vi "Channel Page.vi"(8 "error in (no error)":errorcluster, 11 "Node Ptr":T1 format="%.0x") -> (0 "error out":errorcluster)   [LabVIEW 2009, in "NI-XNET Custom Device.lvlib"]
uses:
  NI-XNET Custom Device.lvlib
  <vilib>/NI VeriStand/Custom Device API/Custom Device Item Ref.ctl
  <vilib>/NI VeriStand/Custom Device API/Get Item Property (Variant).vi
  <vilib>/NI VeriStand/Custom Device API/Custom Device API.lvlib
  Program Files/National Instruments/LabVIEW 2009/resource/objmgr/xnet.rc
panel:
  out "Name":string
  out "Unit":string
  out "Start Bit":u32
  out "Scaling Offset":dbl
  out "Scaling Factor":dbl
  out "Number of Bits":u32
  out "Minimum Value":dbl
  out "Maximum Value":dbl
  out "Default Value":dbl
  out "Data Type":u32(ring) items=["Signed", "Unsigned", "IEEE Float"]
  out "Comment":string
  out "Byte Order":u32(ring) items=["Little Endian", "Big Endian"]
  in  "Header":cluster{"Section Name":string}={"Section Name"="Signal Properties"}
  in  "Delete":bool
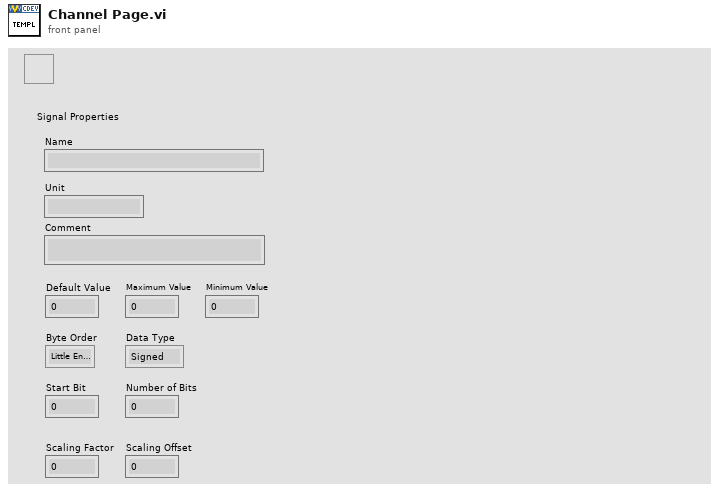
[diagram p1: front panel]
types:
  T1 = typedef "Custom Device API.lvlib/Custom Device Item Ref.ctl" = u64
  T2 = typedef "Custom Device API.lvlib/Custom Device Commands.ctl" = enum16{"Default", "Item renamed", "Shutdown"}
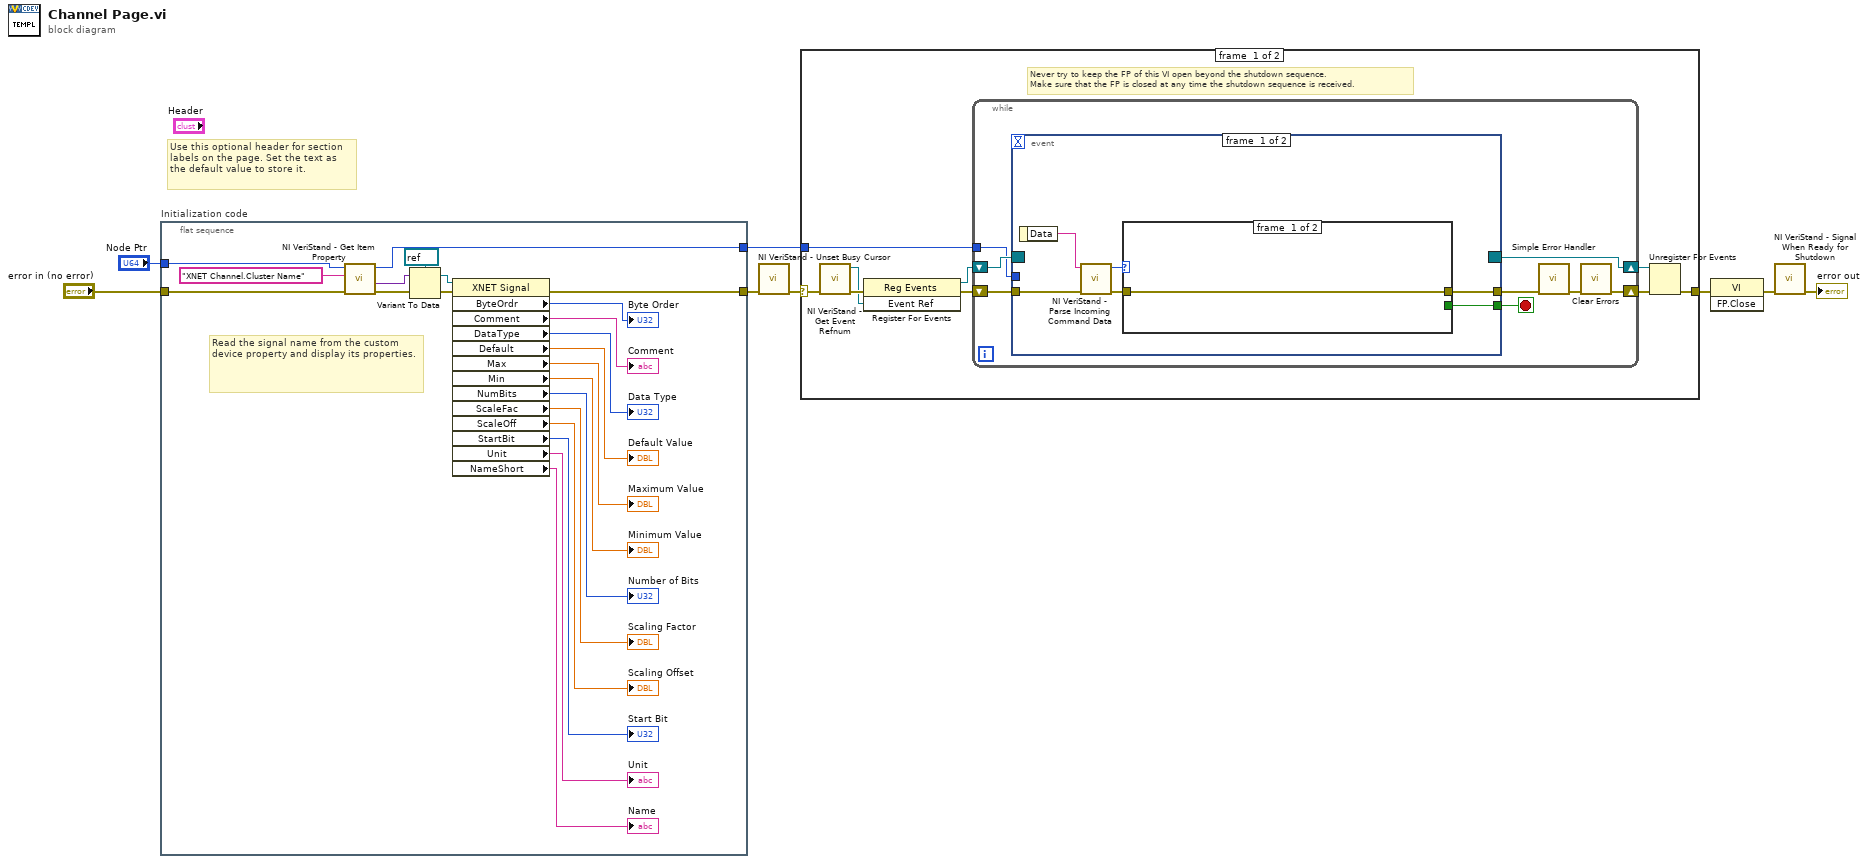
[diagram p0: block diagram]
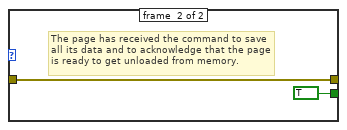
[diagram p2: hidden frame]
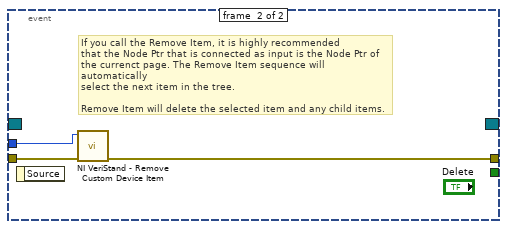
[diagram p3: hidden frame]
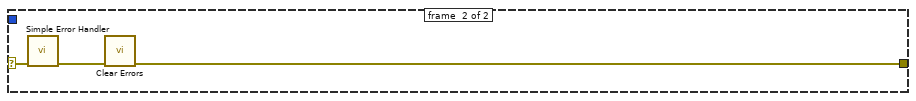
[diagram p4: hidden frame]
diagram:
  # "Use this optional header for section labels on the page. Set the text as the default value to store it."
  n1 = flat-sequence "Initialization code" {
    tunnel: "error in (no error)" -> [w12]
    tunnel: "Node Ptr" -> [w11]
    tunnel: [w24] -> w4
    tunnel: [w10] -> w1
    frame #0 {
      # "Read the signal name from the custom device property and display its properties."
      n2 = call-poly <vilib>:"NI VeriStand - Get Item Property.vi"("error in (no error)"=w12, "Property Name"="XNET Channel.Cluster Name", "Item Ref in"=w11) -> ("error out"=w25:errorcluster, "Value"=w28:variant, "Item Ref out"=w10:T1)  [unwired: 5 in, 1 out]
      n3 = Variant To Data(error in=w25, Variant=w28, type=refnum<k21> refnum ("XNET Signal Constant")) -> (error out=w26:errorcluster, data=w27:refnum<k21>)
      n4 = property class="XNET Signal"(reference=w27, error in=w26) -> (error out=w24:errorcluster, "ByteOrdr"=→"Byte Order":u32, "Comment"=→"Comment":string, "DataType"=→"Data Type":u32, "Default"=→"Default Value":dbl, "Max"=→"Maximum Value":dbl, "Min"=→"Minimum Value":dbl, "NumBits"=→"Number of Bits":u32, "ScaleFac"=→"Scaling Factor":dbl, "ScaleOff"=→"Scaling Offset":dbl, "StartBit"=→"Start Bit":u32, "Unit"=→"Unit":string, "NameShort"=→"Name":string)  [unwired: 1 out]
    }
  }
  n5 = call <vilib>:"NI VeriStand - Unset Busy Cursor.vi"("error in (no error)"=w4) -> ("error out"=w3:errorcluster)  [unwired: 10 out]
  n6 = case shown="No Error" w3 {
    selector: w3 -> [w32 w62]
    tunnel: [w36 w60] -> w8
    tunnel: w1 -> [w31 _]
    frame #0 {
      # "Never try to keep the FP of this VI open beyond the shutdown sequence.\nMake sure that the FP is closed at any time the shutdown sequence is received."
      n7 = call <vilib>:"NI VeriStand - Get Event Refnum.vi"("error in (no error)"=w32) -> ("error out"=w39:errorcluster, "Event Ref"=w35:refnum<user-event>)  [unwired: 9 out]
      n8 = register-events(error in=w39, w35) -> (reference out=w33:refnum<event-registration>, error out=w34:errorcluster)  [unwired: 1 in]
      n9 = while {
        shift-right: [w41] -> w37
        shift-left: w34 -> [w46]
        shift-right: [w47] -> w38
        shift-left: w33 -> [w45]
        tunnel: w31 -> [w40]
        stop <- w44 stop-if-true
        n10 = event shown="[1] \"Delete\": Value Change" {
          selector: w45 -> [_ _]
          dyn-events: [_ _] -> w47
          timeout: _ -> [_ _]
          tunnel: w46 -> [w53 w59]
          tunnel: [w49 _] -> w44
          tunnel: [w48 w58] -> w43
          tunnel: w40 -> [_ w57]
          event #0 {
            n11 = event-data() -> ("Data"=w52:string)  [unwired: 1 out]
            n12 = call <vilib>:"NI VeriStand - Parse Incoming Command Data.vi"("error in (no error)"=w53, "Data"=w52) -> ("error out"=w51:errorcluster, "Action"=w50:T2)  [unwired: 8 out]
            n13 = case shown="\"Shutdown\"" w50 {
              tunnel: w51 -> [w54 w55]
              tunnel: [_ TRUE] -> w49
              tunnel: [w54 w55] -> w48
              frame #0 {
              }
              frame #1 {
                # "The page has received the command to save all its data and to acknowledge that the page is ready to get unloaded from memory."
              }
            }
          }
          event #1 {
            # "If you call the Remove Item, it is highly recommended\nthat the Node Ptr that is connected as input is the Node Ptr of\nthe currenct page. The Remove Item sequence will automatically\nselect the next item in the tree.\n\nRemove Item will delete the selected item and any child items."
            n14 = event-data() -> ()  [unwired: 2 out]
            n15 = call <vilib>:"NI VeriStand - Remove Custom Device Item.vi"("error in (no error)"=w59, "Item Ref in"=w57) -> ("error out"=w58:errorcluster)  [unwired: 1 in, 8 out]
          }
        }
        n16 = call <vilib>:"Simple Error Handler.vi"("error in (no error)"=w43) -> ("error out"=w42:errorcluster)  [unwired: 1 in, 7 out]
        n17 = call <vilib>:"Clear Errors.vi"("error in (no error)"=w42) -> ("error out"=w41:errorcluster)  [unwired: 6 out]
      }
      n18 = Unregister For Events(event registration refnum=w38, error in=w37) -> (error out=w36:errorcluster)
    }
    frame #1 {
      n19 = call <vilib>:"Simple Error Handler.vi"("error in (no error)"=w62) -> ("error out"=w61:errorcluster)  [unwired: 1 in, 7 out]
      n20 = call <vilib>:"Clear Errors.vi"("error in (no error)"=w61) -> ("error out"=w60:errorcluster)  [unwired: 6 out]
    }
  }
  n21 = invoke class="VI" method="FP.Close"(error in=w8) -> (error out=w7:errorcluster)  [unwired: 2 in, 2 out]
  n22 = call <vilib>:"NI VeriStand - Signal When Ready for Shutdown.vi"("error in (no error)"=w7) -> ("error out"=→"error out":errorcluster)  [unwired: 10 out]
